vi "DWE Main3.vi"() -> ()   [LabVIEW 2014]
uses:
  TypeDefs/DWE Errors.ctl
  TypeDefs/DWE Data Info.ctl
  <vilib>/Utility/file.llb/Read From Spreadsheet File (string).vi
panel:
  out "Time array":timestamp[](array[timestamp])
  out "Cluster 2":T2
  out "Day":T2={"Info 1"={"Last time in range?"=TRUE, "Date"="", "Start index"=0}, "Info 2"={"Last time in range?"=TRUE, "Date"="", "Start index"=0}, "Info 3"={"Last time in range?"=TRUE, "Date"="", "Start index"=0}, "Info 4"={"Last time in range?"=TRUE, "Date"="", "Start index"=0}, "info 5"={"Last time in range?"=TRUE, "Date"="", "Start index"=0}, "Info 6"={"Last time in range?"=TRUE, "Date"="", "Start index"=0}, "Info 7"={"Last time in range?"=TRUE, "Date"="", "Start index"=0}, "Info 8"={"Last time in range?"=TRUE, "Date"="", "Start index"=0}, "Info 9"={"Last time in range?"=TRUE, "Date"="", "Start index"=0}, "Info 10"={"Last time in range?"=TRUE, "Date"="", "Start index"=0}}
  in  "Cluster":T2
  out "Iteration":i32
  out "ADC Count":dbl[](array[numeric])
  out "# of rows":i32
  in  "Tab Control":T3(tab)
  out "Current (mA)":cluster{dbl[], dbl[]}(graph)
  out "XY Graph 10":cluster{dbl[], dbl[]}[](graph)
  out "Digital signals":cluster{dbl[], dbl[]}[](graph)
  out "Errors 1":T4
  out "Current (mA) 2":cluster{dbl[], dbl[]}(graph)
  out "XY Graph 11":cluster{dbl[], dbl[]}[](graph)
  out "Digital signals 3":cluster{dbl[], dbl[]}[](graph)
  out "Errors 2":T4
  out "Digital signals 2":cluster{dbl[], dbl[]}[](graph)
  out "Current (mA) 3":cluster{dbl[], dbl[]}(graph)
  out "XY Graph 12":cluster{dbl[], dbl[]}[](graph)
  out "Errors 3":T4
  out "Digital signals 4":cluster{dbl[], dbl[]}[](graph)
  out "Current (mA) 4":cluster{dbl[], dbl[]}(graph)
  out "XY Graph 13":cluster{dbl[], dbl[]}[](graph)
  out "Errors 11":T4
  out "Digital signals 5":cluster{dbl[], dbl[]}[](graph)
  out "Current (mA) 5":cluster{dbl[], dbl[]}(graph)
  out "XY Graph 14":cluster{dbl[], dbl[]}[](graph)
  out "Errors 4":T4
  out "Digital signals 6":cluster{dbl[], dbl[]}[](graph)
  out "Current (mA) 6":cluster{dbl[], dbl[]}(graph)
  out "XY Graph 15":cluster{dbl[], dbl[]}[](graph)
  out "Errors 5":T4
  out "Digital signals 7":cluster{dbl[], dbl[]}[](graph)
  out "Current (mA) 7":cluster{dbl[], dbl[]}(graph)
  out "XY Graph 16":cluster{dbl[], dbl[]}[](graph)
  out "Errors 6":T4
  out "Digital signals 8":cluster{dbl[], dbl[]}[](graph)
  out "Current (mA) 8":cluster{dbl[], dbl[]}(graph)
  out "XY Graph 17":cluster{dbl[], dbl[]}[](graph)
  out "Errors 7":T4
  out "Digital signals 9":cluster{dbl[], dbl[]}[](graph)
  out "Current (mA) 9":cluster{dbl[], dbl[]}(graph)
  out "XY Graph 18":cluster{dbl[], dbl[]}[](graph)
  out "Errors 8":T4
  out "Digital signals 10":cluster{dbl[], dbl[]}[](graph)
  out "Current (mA) 10":cluster{dbl[], dbl[]}(graph)
  out "XY Graph 19":cluster{dbl[], dbl[]}[](graph)
  out "Errors 9":T4
  out "subarray":string[][](array[string])
  out "subarray 3":string[](array[string])
  in  "stop":bool
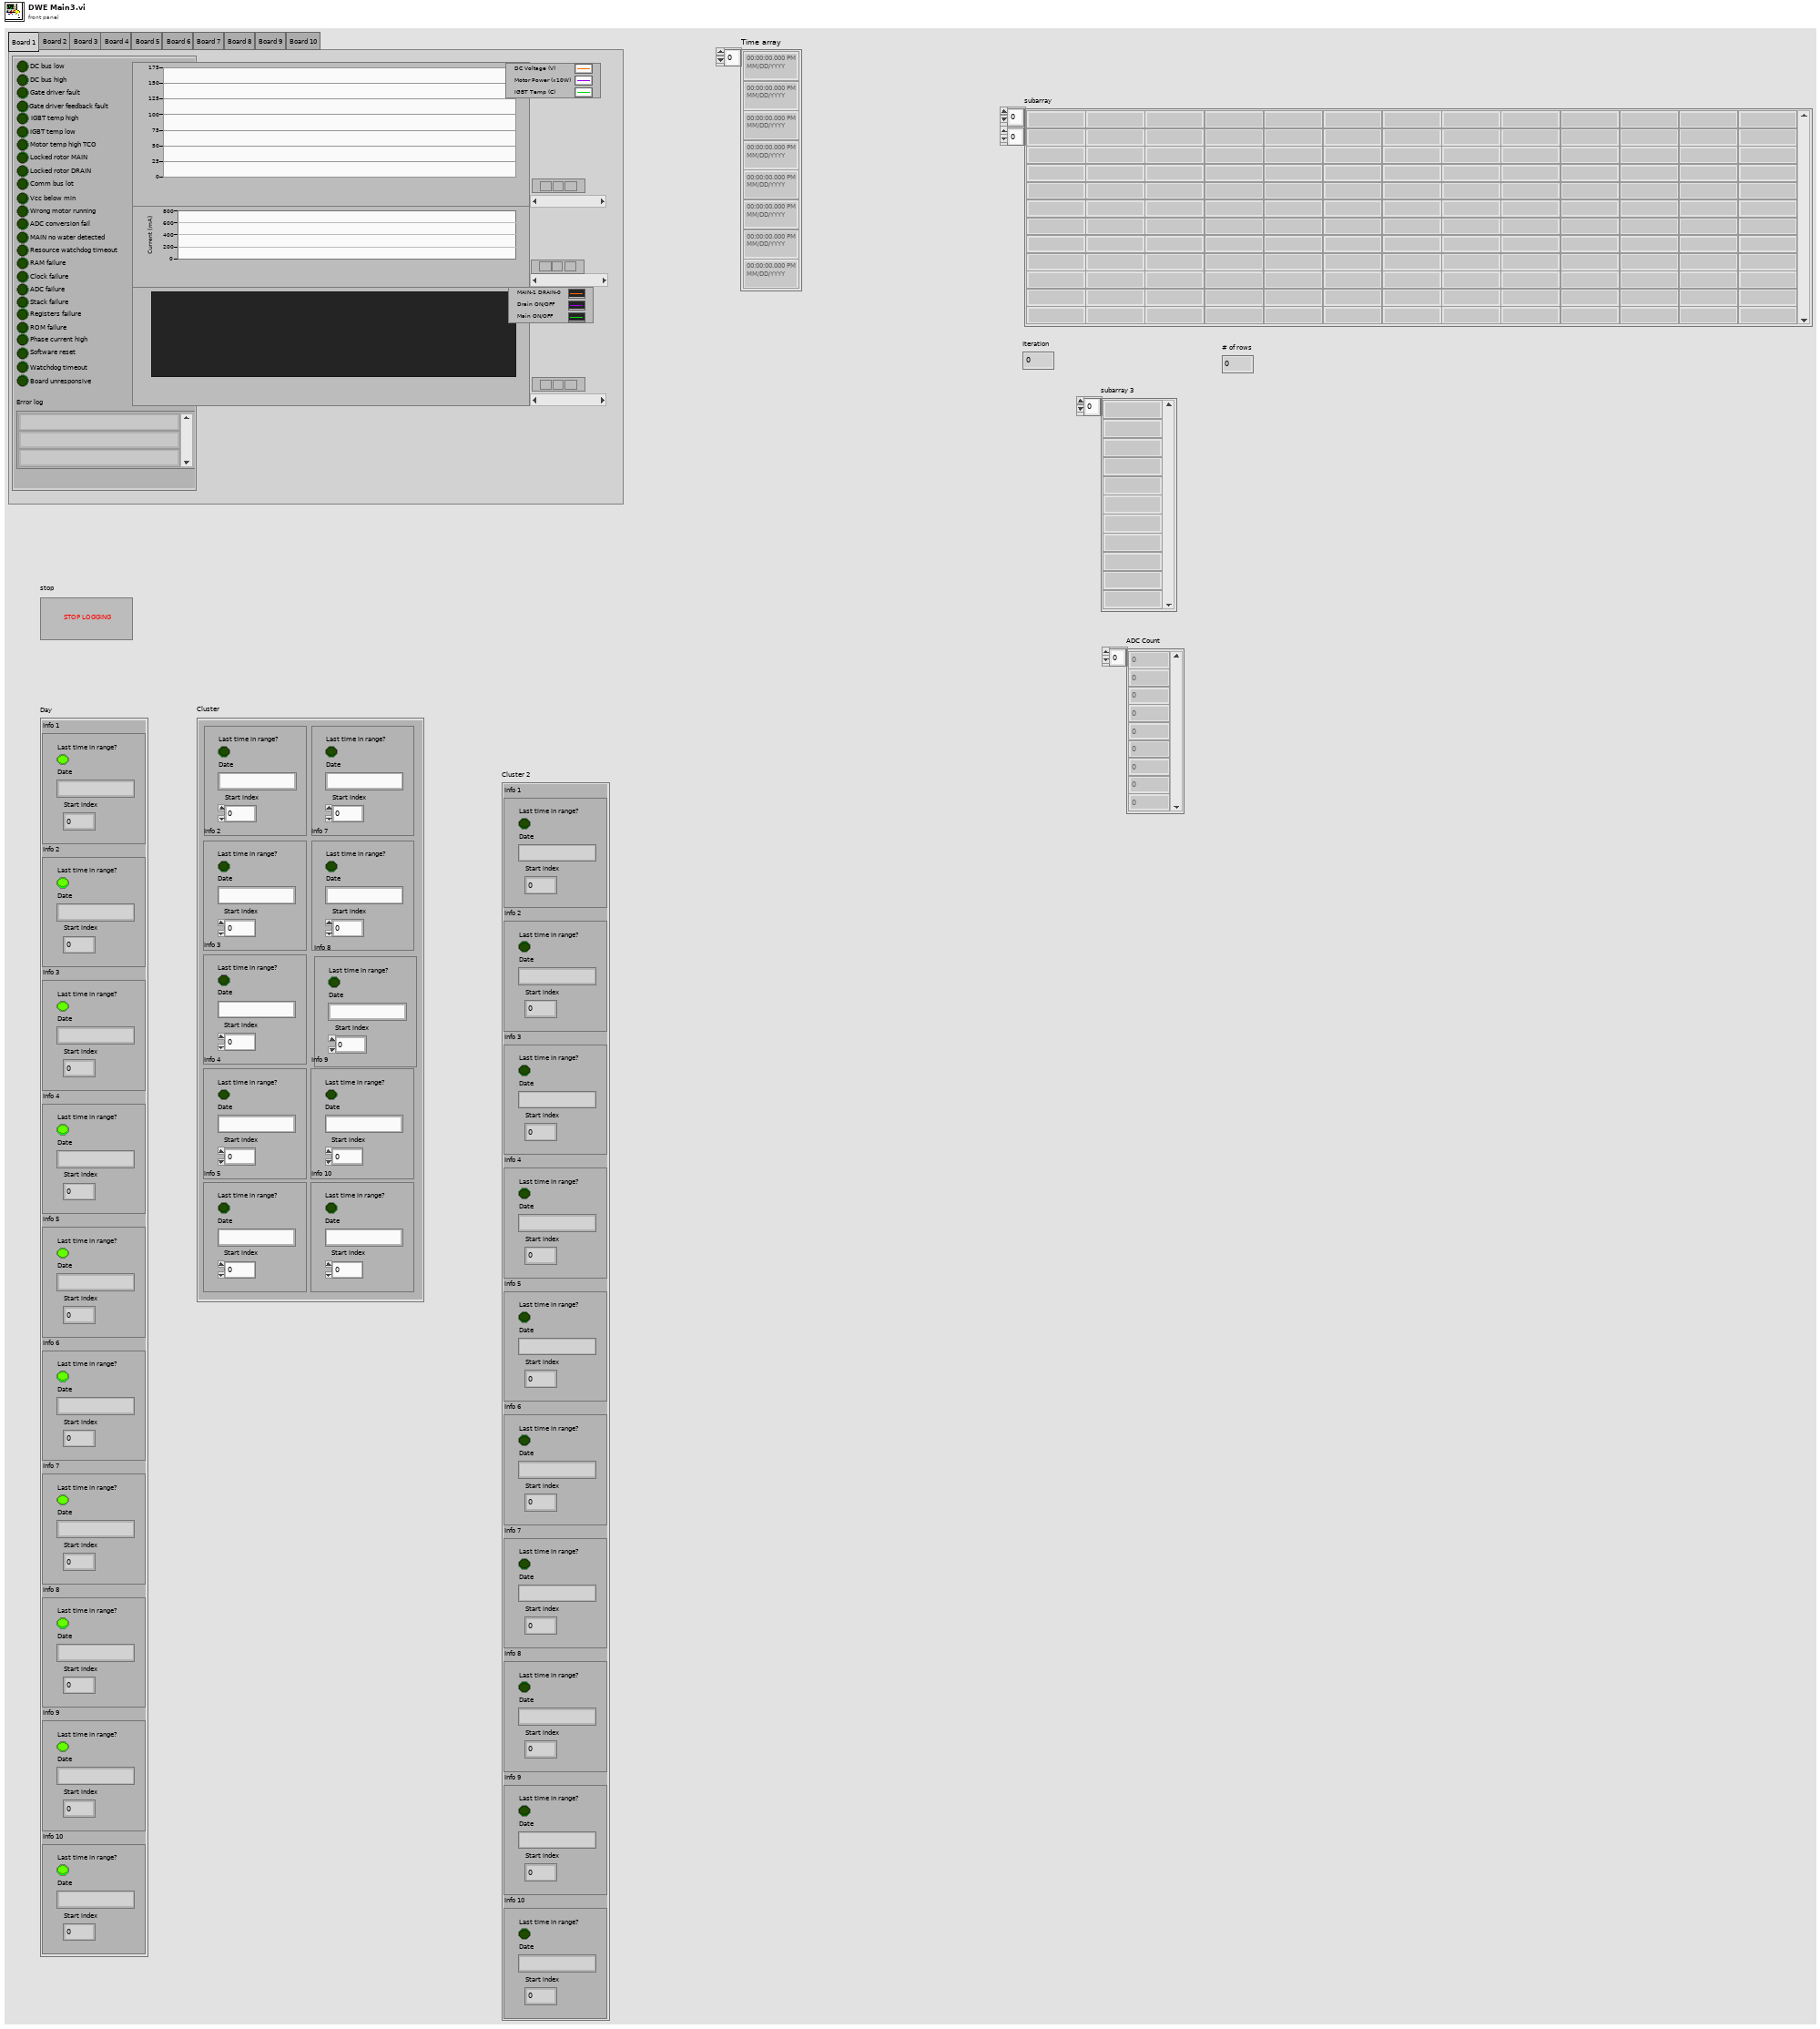
[diagram p1: front panel]
types:
  T1 = typedef "DWE Data Info.ctl" = cluster{"Last time in range?":bool, "Date":string, "Start index":i32}
  T2 = cluster{"Info 1":T1, "Info 2":T1, "Info 3":T1, "Info 4":T1, "info 5":T1, "Info 6":T1, "Info 7":T1, "Info 8":T1, "Info 9":T1, "Info 10":T1}
  T3 = enum32{"Board 1", "Board 2", "Board 3", "Board 4", "Board 5", "Board 6", "Board 7", "Board 8", "Board 9", "Board 10"}
  T4 = typedef "DWE Errors.ctl" = cluster{"DC bus low":bool, "DC bus high":bool, "Gate driver fault":bool, "Gate driver feedback fault":bool, "IGBT temp high":bool, "IGBT temp low":bool, "Motor temp high TCO":bool, "Locked rotor MAIN":bool, "Locked rotor DRAIN":bool, "Comm bus lot":bool, "Vcc below min":bool, "Wrong motor running":bool, "ADC conversion fail":bool, "MAIN no water detected":bool, "Resource watchdog timeout":bool, "RAM failure":bool, "Clock failure":bool, "ADC failure":bool, "Stack failure":bool, "Registers failure":bool, "ROM failure":bool, "Phase current high":bool, "Software reset":bool, "Watchdog timeout":bool, "Error log":string[], "Board unresponsive":bool}
  T5 = cluster{"01 File Path":path, "02 File Path":path, "03 File Path":path, "04 File Path":path, "05 File Path":path, "06 File Path":path, "07 File Path":path, "08 File Path":path, "09 File Path":path, "10 File Path":path}
  T6 = cluster{"Last time in range?":bool, "date/time string":string, "Start index":i32}
  T7 = cluster{"DC Bus Voltage":dbl, "Current RMS":dbl, "Motor Power":dbl, "IGBT Temp":u16, "Motor Type":u16, "Motor Power Sign":string, "Relay Position":u16, "ADC Count":dbl, "Recirculation Motor ON/OFF":u16, "Drain Motor ON/OFF":u16}
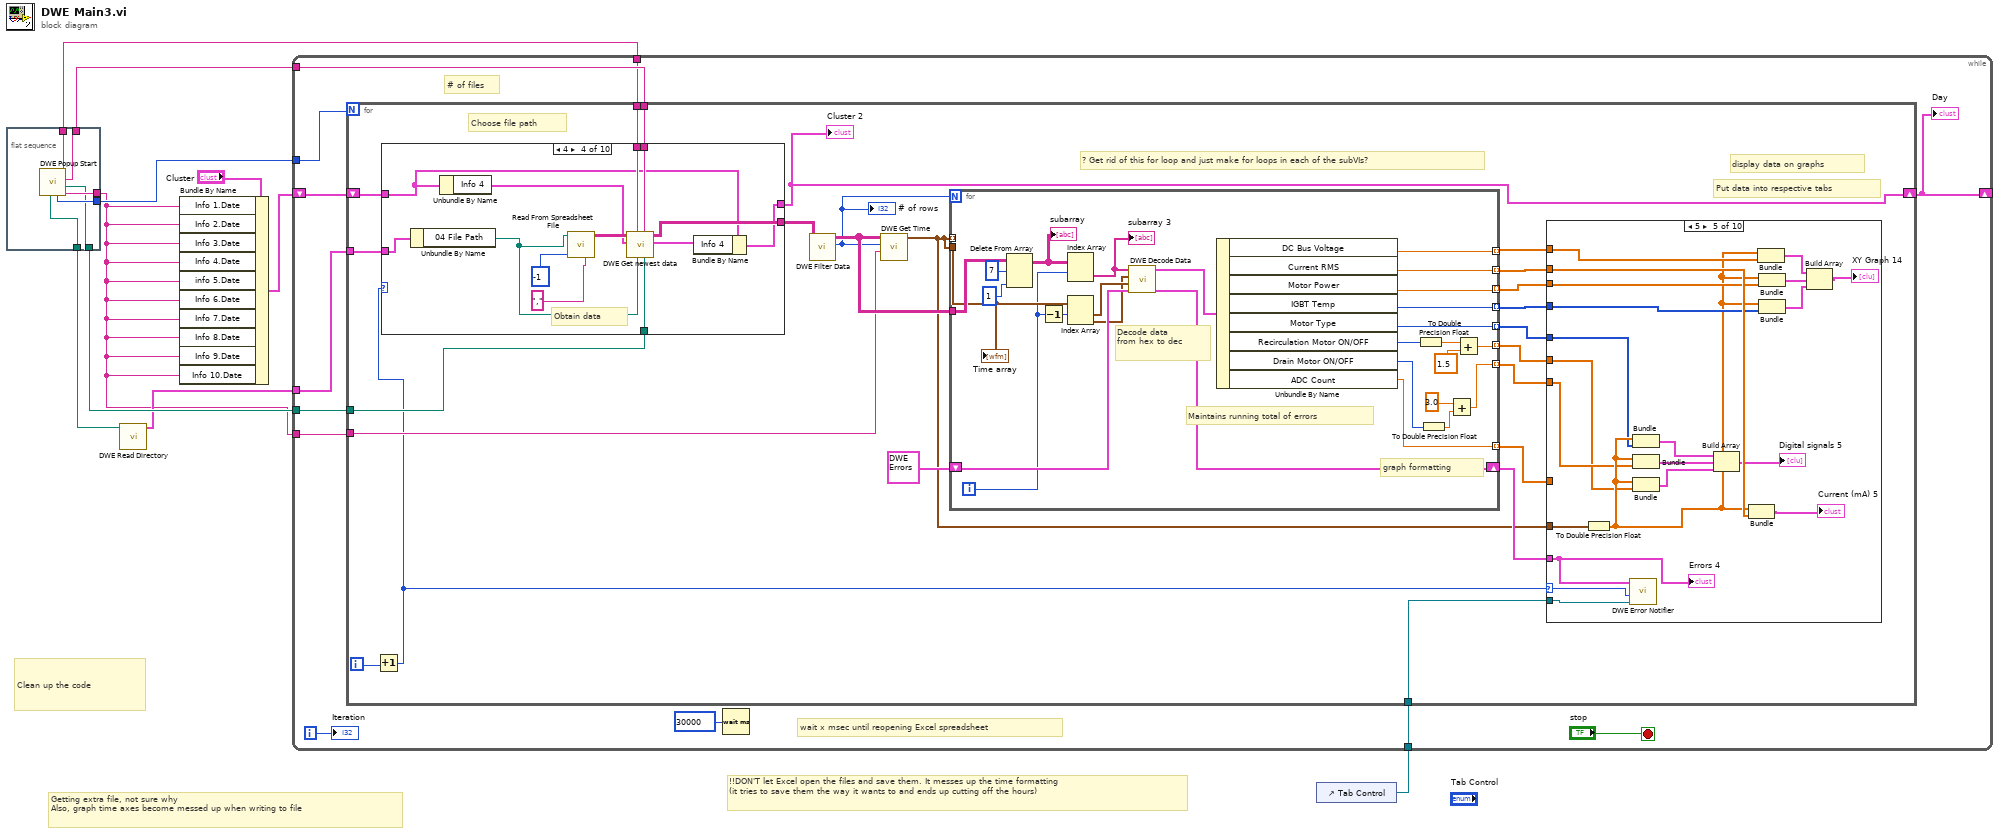
[diagram p0: block diagram]
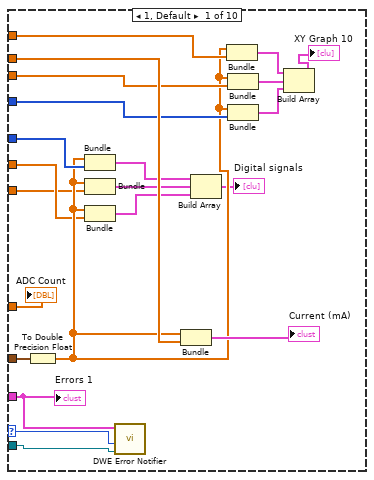
[diagram p2: hidden frame]
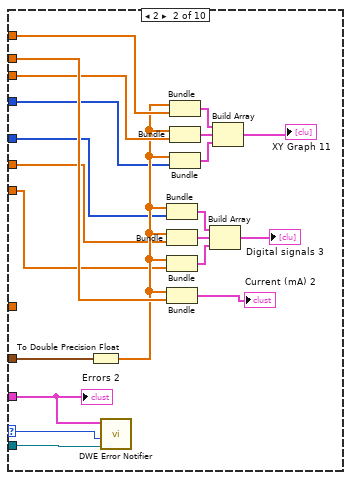
[diagram p3: hidden frame]
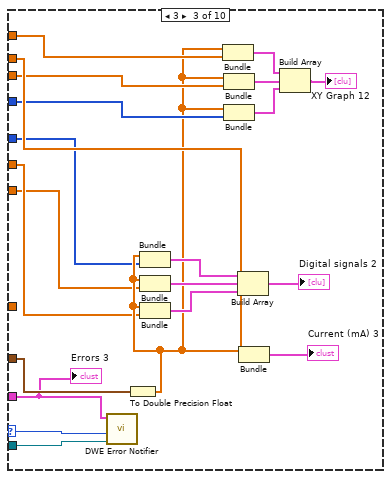
[diagram p4: hidden frame]
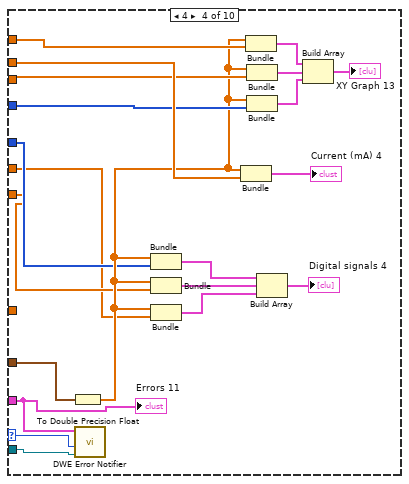
[diagram p5: hidden frame]
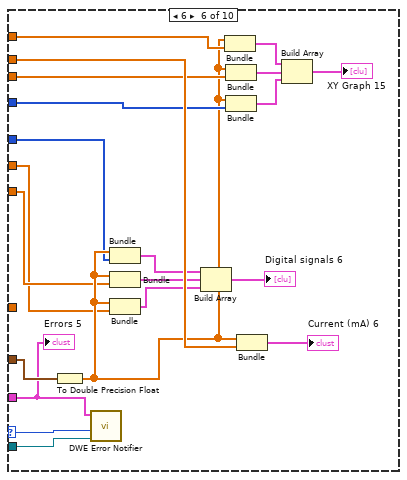
[diagram p6: hidden frame]
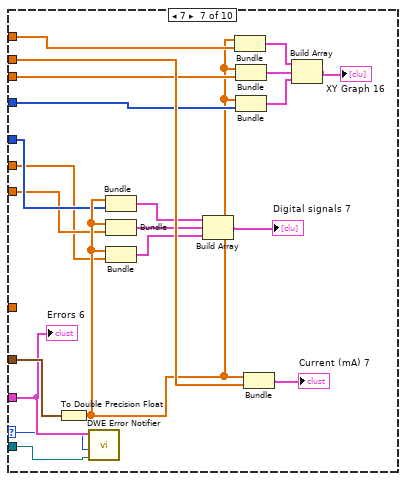
[diagram p7: hidden frame]
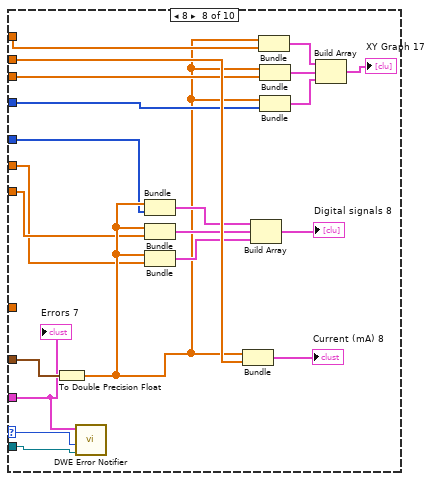
[diagram p8: hidden frame]
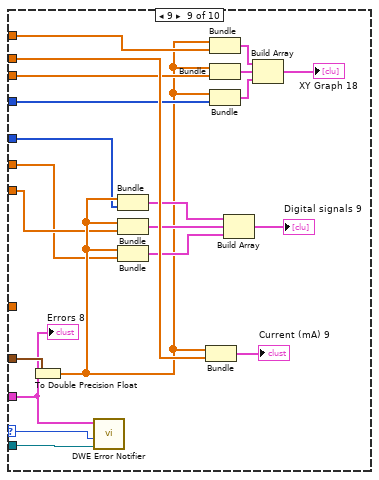
[diagram p9: hidden frame]
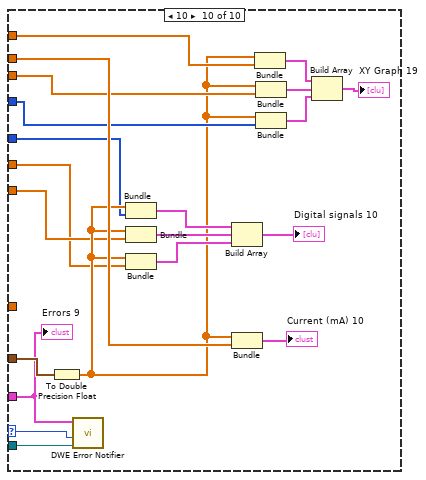
[diagram p10: hidden frame]
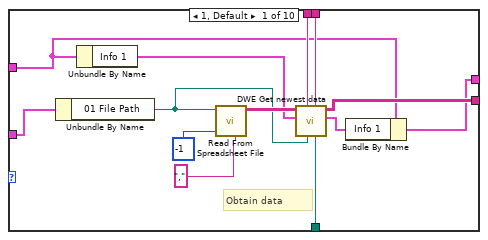
[diagram p11: hidden frame]
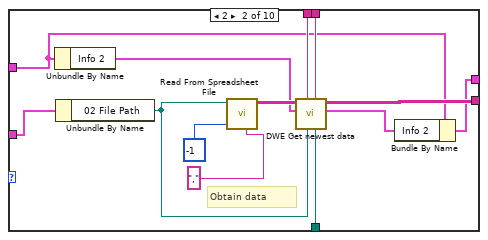
[diagram p12: hidden frame]
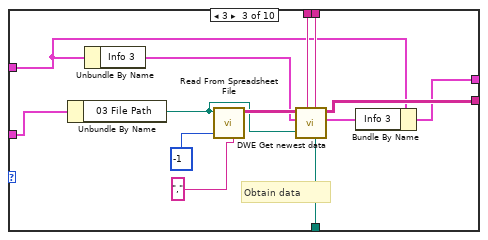
[diagram p13: hidden frame]
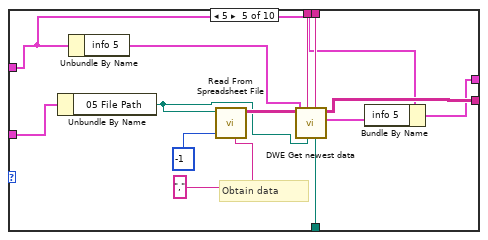
[diagram p14: hidden frame]
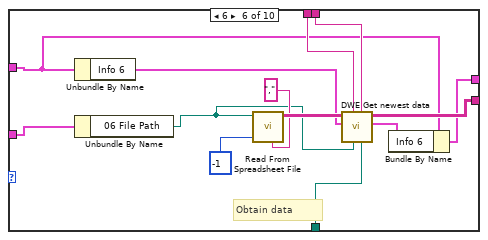
[diagram p15: hidden frame]
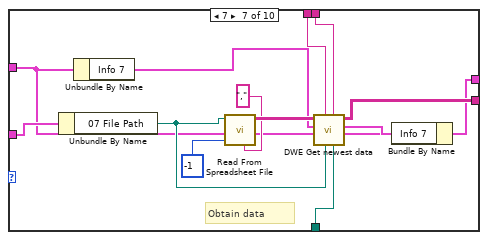
[diagram p16: hidden frame]
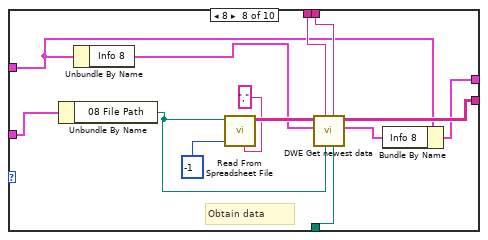
[diagram p17: hidden frame]
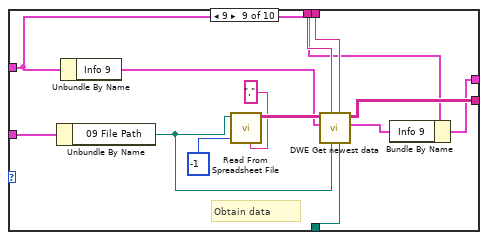
[diagram p18: hidden frame]
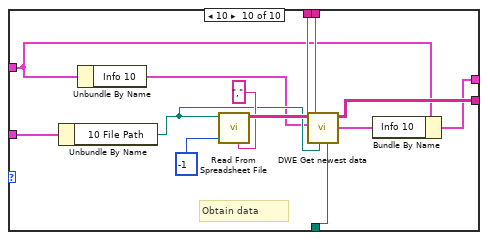
[diagram p19: hidden frame]
diagram:
  # "Getting extra file, not sure why\nAlso, graph time axes become messed up when writing to file"
  # "Clean up the code"
  # "!!DON'T let Excel open the files and save them. It messes up the time formatting \n(it tries to save them the way it wants to and ends up cutting off the hours)"
  n1 = flat-sequence {
    tunnel: [w16] -> w2
    tunnel: [w15] -> w8
    tunnel: [w14] -> w3
    tunnel: [w13] -> w7
    tunnel: [w12] -> w6
    tunnel: [w11] -> w5
    frame #0 {
      n2 = call "DWE Popup Start.vi"() -> ("Date Laundry.NET\nstarted (MM_DD) 2"=w16:string, "Folder to store data sets 2"=w13:path, "End time save 2"=w12:string, "Start time save 2"=w11:string, "# of Files 2"=w15:i32, "File directory 2"=w14:path)  [unwired: 6 in]
    }
  }
  n3 = call "DWE Read Directory.vi"("path"=w3) -> ("Laundry.NET \nfile paths 3"=w4:T5)  [unwired: 10 in]
  n4 = Bundle By Name(cluster="Cluster", "Info 1.Date"=w2, "Info 2.Date"=w2, "Info 3.Date"=w2, "Info 4.Date"=w2, "info 5.Date"=w2, "Info 6.Date"=w2, "Info 7.Date"=w2, "Info 8.Date"=w2, "Info 9.Date"=w2, "Info 10.Date"=w2) -> (w9:T2)
  n5 = control-ref of="Tab Control"() -> (w1:refnum<vi>)
  n6 = while {
    shift-right: [w25] -> _
    shift-left: w9 -> [w19]
    tunnel: w8 -> [w24]
    tunnel: w4 -> [w23]
    tunnel: w7 -> [w22]
    tunnel: w6 -> [w21]
    tunnel: w5 -> [w20]
    tunnel: w2 -> [w18]
    tunnel: w1 -> [w17]
    i -> [w26]
    stop <- "stop" stop-if-true
    # "# of files"
    # "wait x msec until reopening Excel spreadsheet"
    n7 = for {
      N: w24 -> [_]
      tunnel: w23 -> [w52]
      tunnel: w21 -> [w39]
      tunnel: w22 -> [w37]
      tunnel: w20 -> [w36]
      shift-right: [w38] -> w25
      shift-left: w19 -> [w35]
      tunnel: w18 -> [w33]
      tunnel: w17 -> [w32]
      i -> [w31]
      # "? Get rid of this for loop and just make for loops in each of the subVIs?"
      # "display data on graphs"
      # "Put data into respective tabs"
      # "Choose file path"
      n8 = Increment(x=w31) -> (x+1=w30:i32)
      n9 = case shown="4" w30 {
        tunnel: w52 -> [w276 w289 w302 w315 w328 w341 w354 w367 w380 w393]
        tunnel: [w272 w285 w298 w311 w324 w337 w350 w363 w376 w389] -> w40
        tunnel: w37 -> [w270 w281 w294 w307 w320 w335 w346 w359 w372 w385]
        tunnel: w36 -> [w269 w284 w297 w310 w323 w334 w349 w362 w375 w388]
        tunnel: w39 -> [w268 w283 w296 w309 w322 w333 w348 w361 w374 w387]
        tunnel: w35 -> [w265 w278 w292 w304 w317 w330 w343 w356 w369 w383]
        tunnel: [w264 w277 w290 w303 w316 w329 w342 w355 w368 w381] -> w38
        frame 1, Default {
          # "Obtain data"
          n10 = Unbundle By Name(w276) -> ("01 File Path"=w271:path)
          n11 = Unbundle By Name(w265) -> ("Info 1"=w267:T1)
          n12 = call-poly <vilib>:"Read From Spreadsheet File.vi"("delimiter (\\t)"="," ("delimiter (\\t)"), "number of rows (all:-1)"=-1, "file path (dialog if empty)"=w271) -> ("all rows"=w275:string[][])  [unwired: 4 in, 4 out]
          n13 = call "DWE Get newest data.vi"("target path"=w270, "End time"=w268, "source path"=w271, "Start time"=w269, "Previous info"=w267, "all rows"=w275) -> ("New Info"=w266:T6, "newest rows"=w272:string[][])  [unwired: 4 in]
          n14 = Bundle By Name(cluster=w265, "Info 1"=w266) -> (w264:T2)
        }
        frame 2 {
          # "Obtain data"
          n15 = Unbundle By Name(w278) -> ("Info 2"=w280:T1)
          n16 = Unbundle By Name(w289) -> ("02 File Path"=w282:path)
          n17 = call-poly <vilib>:"Read From Spreadsheet File.vi"("delimiter (\\t)"="," ("delimiter (\\t)"), "number of rows (all:-1)"=-1, "file path (dialog if empty)"=w282) -> ("all rows"=w288:string[][])  [unwired: 4 in, 4 out]
          n18 = call "DWE Get newest data.vi"("target path"=w281, "End time"=w283, "source path"=w282, "Start time"=w284, "Previous info"=w280, "all rows"=w288) -> ("New Info"=w279:T6, "newest rows"=w285:string[][])  [unwired: 4 in]
          n19 = Bundle By Name(cluster=w278, "Info 2"=w279) -> (w277:T2)
        }
        frame 3 {
          # "Obtain data"
          n20 = Unbundle By Name(w302) -> ("03 File Path"=w295:path)
          n21 = Unbundle By Name(w292) -> ("Info 3"=w293:T1)
          n22 = call-poly <vilib>:"Read From Spreadsheet File.vi"("delimiter (\\t)"="," ("delimiter (\\t)"), "number of rows (all:-1)"=-1, "file path (dialog if empty)"=w295) -> ("all rows"=w301:string[][])  [unwired: 4 in, 4 out]
          n23 = call "DWE Get newest data.vi"("target path"=w294, "End time"=w296, "source path"=w295, "Start time"=w297, "Previous info"=w293, "all rows"=w301) -> ("New Info"=w291:T6, "newest rows"=w298:string[][])  [unwired: 4 in]
          n24 = Bundle By Name(cluster=w292, "Info 3"=w291) -> (w290:T2)
        }
        frame 4 {
          # "Obtain data"
          n25 = Unbundle By Name(w315) -> ("04 File Path"=w308:path)
          n26 = Unbundle By Name(w304) -> ("Info 4"=w306:T1)
          n27 = call-poly <vilib>:"Read From Spreadsheet File.vi"("delimiter (\\t)"="," ("delimiter (\\t)"), "number of rows (all:-1)"=-1, "file path (dialog if empty)"=w308) -> ("all rows"=w314:string[][])  [unwired: 4 in, 4 out]
          n28 = call "DWE Get newest data.vi"("target path"=w307, "End time"=w309, "source path"=w308, "Start time"=w310, "Previous info"=w306, "all rows"=w314) -> ("New Info"=w305:T6, "newest rows"=w311:string[][])  [unwired: 4 in]
          n29 = Bundle By Name(cluster=w304, "Info 4"=w305) -> (w303:T2)
        }
        frame 5 {
          # "Obtain data"
          n30 = Unbundle By Name(w328) -> ("05 File Path"=w321:path)
          n31 = Unbundle By Name(w317) -> ("info 5"=w319:T1)
          n32 = call-poly <vilib>:"Read From Spreadsheet File.vi"("delimiter (\\t)"="," ("delimiter (\\t)"), "number of rows (all:-1)"=-1, "file path (dialog if empty)"=w321) -> ("all rows"=w327:string[][])  [unwired: 4 in, 4 out]
          n33 = call "DWE Get newest data.vi"("target path"=w320, "End time"=w322, "source path"=w321, "Start time"=w323, "Previous info"=w319, "all rows"=w327) -> ("New Info"=w318:T6, "newest rows"=w324:string[][])  [unwired: 4 in]
          n34 = Bundle By Name(cluster=w317, "info 5"=w318) -> (w316:T2)
        }
        frame 6 {
          # "Obtain data"
          n35 = Unbundle By Name(w330) -> ("Info 6"=w332:T1)
          n36 = Unbundle By Name(w341) -> ("06 File Path"=w336:path)
          n37 = call-poly <vilib>:"Read From Spreadsheet File.vi"("delimiter (\\t)"="," ("delimiter (\\t)"), "number of rows (all:-1)"=-1, "file path (dialog if empty)"=w336) -> ("all rows"=w340:string[][])  [unwired: 4 in, 4 out]
          n38 = call "DWE Get newest data.vi"("target path"=w335, "End time"=w333, "source path"=w336, "Start time"=w334, "Previous info"=w332, "all rows"=w340) -> ("New Info"=w331:T6, "newest rows"=w337:string[][])  [unwired: 4 in]
          n39 = Bundle By Name(cluster=w330, "Info 6"=w331) -> (w329:T2)
        }
        frame 7 {
          # "Obtain data"
          n40 = Unbundle By Name(w354) -> ("07 File Path"=w347:path)
          n41 = Unbundle By Name(w343) -> ("Info 7"=w345:T1)
          n42 = call-poly <vilib>:"Read From Spreadsheet File.vi"("delimiter (\\t)"="," ("delimiter (\\t)"), "number of rows (all:-1)"=-1, "file path (dialog if empty)"=w347) -> ("all rows"=w353:string[][])  [unwired: 4 in, 4 out]
          n43 = call "DWE Get newest data.vi"("target path"=w346, "End time"=w348, "source path"=w347, "Start time"=w349, "Previous info"=w345, "all rows"=w353) -> ("New Info"=w344:T6, "newest rows"=w350:string[][])  [unwired: 4 in]
          n44 = Bundle By Name(cluster=w343, "Info 7"=w344) -> (w342:T2)
        }
        frame 8 {
          # "Obtain data"
          n45 = Unbundle By Name(w367) -> ("08 File Path"=w360:path)
          n46 = Unbundle By Name(w356) -> ("Info 8"=w358:T1)
          n47 = call-poly <vilib>:"Read From Spreadsheet File.vi"("delimiter (\\t)"="," ("delimiter (\\t)"), "number of rows (all:-1)"=-1, "file path (dialog if empty)"=w360) -> ("all rows"=w366:string[][])  [unwired: 4 in, 4 out]
          n48 = call "DWE Get newest data.vi"("target path"=w359, "End time"=w361, "source path"=w360, "Start time"=w362, "Previous info"=w358, "all rows"=w366) -> ("New Info"=w357:T6, "newest rows"=w363:string[][])  [unwired: 4 in]
          n49 = Bundle By Name(cluster=w356, "Info 8"=w357) -> (w355:T2)
        }
        frame 9 {
          # "Obtain data"
          n50 = Unbundle By Name(w380) -> ("09 File Path"=w373:path)
          n51 = Unbundle By Name(w369) -> ("Info 9"=w371:T1)
          n52 = call-poly <vilib>:"Read From Spreadsheet File.vi"("delimiter (\\t)"="," ("delimiter (\\t)"), "number of rows (all:-1)"=-1, "file path (dialog if empty)"=w373) -> ("all rows"=w379:string[][])  [unwired: 4 in, 4 out]
          n53 = call "DWE Get newest data.vi"("target path"=w372, "End time"=w374, "source path"=w373, "Start time"=w375, "Previous info"=w371, "all rows"=w379) -> ("New Info"=w370:T6, "newest rows"=w376:string[][])  [unwired: 4 in]
          n54 = Bundle By Name(cluster=w369, "Info 9"=w370) -> (w368:T2)
        }
        frame 10 {
          # "Obtain data"
          n55 = Unbundle By Name(w393) -> ("10 File Path"=w386:path)
          n56 = Unbundle By Name(w383) -> ("Info 10"=w384:T1)
          n57 = call-poly <vilib>:"Read From Spreadsheet File.vi"("delimiter (\\t)"="," ("delimiter (\\t)"), "number of rows (all:-1)"=-1, "file path (dialog if empty)"=w386) -> ("all rows"=w392:string[][])  [unwired: 4 in, 4 out]
          n58 = call "DWE Get newest data.vi"("target path"=w385, "End time"=w387, "source path"=w386, "Start time"=w388, "Previous info"=w384, "all rows"=w392) -> ("New Info"=w382:T6, "newest rows"=w389:string[][])  [unwired: 4 in]
          n59 = Bundle By Name(cluster=w383, "Info 10"=w382) -> (w381:T2)
        }
      }
      "Cluster 2" <- w38
      n60 = call "DWE Filter Data.vi"("All Rows"=w40) -> ("element"=w34:i32, "new array"=w45:string[][])  [unwired: 9 in]
      "# of rows" <- w34
      n61 = call "DWE Get Time.vi"("Date"=w33, "# of rows"=w34, "Data row"=w45) -> ("Time array"=w29:timestamp[])  [unwired: 8 in]
      n62 = for {
        N: w34 -> [_]
        tunnel: [w420] -> w49 mode=indexing
        tunnel: [w419] -> w51 mode=indexing
        tunnel: [w418] -> w50 mode=indexing
        tunnel: [w417] -> w48 mode=indexing
        tunnel: [w416] -> w47 mode=indexing
        shift-right: [w403] -> w46
        shift-left: T4 {"DC bus low"=FALSE, "DC bus high"=FALSE, "Gate driver fault"=FALSE, "Gate driver feedback fault"=FALSE, "IGBT temp high"=FALSE, "IGBT temp low"=FALSE, "Motor temp high TCO"=FALSE, "Locked rotor MAIN"=FALSE, "Locked rotor DRAIN"=FALSE, "Comm bus lot"=FALSE, "Vcc below min"=FALSE, "Wrong motor running"=FALSE, "ADC conversion fail"=FALSE, "MAIN no water detected"=FALSE, "Resource watchdog timeout"=FALSE, "RAM failure"=FALSE, "Clock failure"=FALSE, "ADC failure"=FALSE, "Stack failure"=FALSE, "Registers failure"=FALSE, "ROM failure"=FALSE, "Phase current high"=FALSE, "Software reset"=FALSE, "Watchdog timeout"=FALSE, "Error log"=[], "Board unresponsive"=FALSE} ("Errors Out") -> [w415]
        tunnel: w45 -> [w402]
        tunnel: [w412] -> w42 mode=indexing
        tunnel: [w411] -> w43 mode=indexing
        tunnel: [w404] -> w41 mode=indexing
        tunnel: w29 -> [_] mode=indexing
        tunnel: w29 -> [w398]
        i -> [w394]
        # "graph formatting"
        # "Maintains running total of errors"
        # "Decode data\nfrom hex to dec"
        n63 = Delete From Array(array=w402, length=7, index (col)=1 ("disabled index (col)")) -> (array with subset deleted=w399:string[][])  [unwired: 1 in, 1 out]
        "subarray" <- w399
        n64 = Decrement(x=w394) -> (x-1=w395:i32)
        n65 = Index Array(array=w399, index (row)=w394) -> (element=w413:string[])  [unwired: 1 in]
        "subarray 3" <- w413
        n66 = Index Array(array=w398, index #1=w395) -> (element #1=w397:timestamp, element #2=w396:timestamp)  [unwired: 1 in]
        n67 = call "DWE Decode Data.vi"("Errors In"=w415, "Prev time stamp"=w397, "Time Stamp"=w396, "Data Array"=w413) -> ("Errors Out"=w403:T4, "logData Out"=w414:T7)  [unwired: 6 in]
        n68 = Unbundle By Name(w414) -> ("DC Bus Voltage"=w420:dbl, "Current RMS"=w419:dbl, "Motor Power"=w418:dbl, "IGBT Temp"=w417:u16, "Motor Type"=w416:u16, "Recirculation Motor ON/OFF"=w410:u16, "Drain Motor ON/OFF"=w407:u16, "ADC Count"=w404:dbl)
        n69 = To Double Precision Float(number=w410) -> (double precision float=w409:dbl)
        n70 = To Double Precision Float(number=w407) -> (double precision float=w406:dbl)
        n71 = Add(x=3.0, y=w406) -> (x+y=w411:dbl)
        n72 = Add(x=w409, y=1.5) -> (x+y=w412:dbl)
        "Time array" <- w398
      }
      n73 = case shown="5" w30 {
        selector: w30 -> [w54 w76 w97 w118 w140 w160 w181 w202 w223 w244]
        tunnel: w51 -> [w74 w94 w115 w136 w157 w178 w199 w220 w241 w262]
        tunnel: w50 -> [w66 w89 w110 w130 w152 w173 w194 w215 w237 w260]
        tunnel: w49 -> [w67 w90 w111 w132 w153 w174 w195 w216 w238 w261]
        tunnel: w48 -> [w65 w84 w109 w131 w151 w172 w193 w214 w236 w259]
        tunnel: w47 -> [w64 w78 w104 w125 w146 w167 w188 w209 w230 w251]
        tunnel: w46 -> [w55 w77 w98 w119 w141 w161 w182 w203 w224 w245]
        tunnel: w29 -> [w73 w95 w116 w137 w158 w179 w200 w221 w242 w263]
        tunnel: w42 -> [w62 w83 w103 w123 w144 w165 w186 w207 w228 w249]
        tunnel: w43 -> [w61 w82 w102 w124 w145 w166 w187 w208 w229 w250]
        tunnel: w41 -> [w56 _ _ _ _ _ _ _ _ _]
        tunnel: w32 -> [w53 w75 w96 w117 w139 w159 w180 w201 w222 w243]
        frame 1, Default {
          n74 = To Double Precision Float(number=w73) -> (double precision float=w63:dbl[])
          n75 = Bundle(w63, w64) -> (w60:cluster{dbl[], u16[]})  [unwired: 1 in]
          n76 = Bundle(w63, w61) -> (w58:cluster{dbl[], dbl[]})  [unwired: 1 in]
          n77 = Bundle(w63, w62) -> (w57:cluster{dbl[], dbl[]})  [unwired: 1 in]
          n78 = call "DWE Error Notifier.vi"("Tab Control 3"=w53, "Tab num"=w54, "Errors 1"=w55) -> ()  [unwired: 8 in, 1 out]
          n79 = Bundle(w63, w74) -> (→"Current (mA)":cluster{dbl[], dbl[]})  [unwired: 1 in]
          n80 = Build Array(w60, w58, w57) -> (→"Digital signals":cluster{dbl[], dbl[]}[])
          n81 = Bundle(w63, w67) -> (w71:cluster{dbl[], dbl[]})  [unwired: 1 in]
          n82 = Bundle(w63, w66) -> (w70:cluster{dbl[], dbl[]})  [unwired: 1 in]
          n83 = Bundle(w63, w65) -> (w69:cluster{dbl[], u16[]})  [unwired: 1 in]
          n84 = Build Array(w71, w70, w69) -> (→"XY Graph 10":cluster{dbl[], dbl[]}[])
          "Errors 1" <- w55
          "ADC Count" <- w56
        }
        frame 2 {
          n85 = To Double Precision Float(number=w95) -> (double precision float=w85:dbl[])
          n86 = call "DWE Error Notifier.vi"("Tab Control 3"=w75, "Tab num"=w76, "Errors 1"=w77) -> ()  [unwired: 8 in, 1 out]
          n87 = Bundle(w85, w78) -> (w88:cluster{dbl[], u16[]})  [unwired: 1 in]
          n88 = Bundle(w85, w83) -> (w87:cluster{dbl[], dbl[]})  [unwired: 1 in]
          n89 = Bundle(w85, w82) -> (w86:cluster{dbl[], dbl[]})  [unwired: 1 in]
          n90 = Bundle(w85, w94) -> (→"Current (mA) 2":cluster{dbl[], dbl[]})  [unwired: 1 in]
          n91 = Bundle(w85, w90) -> (w93:cluster{dbl[], dbl[]})  [unwired: 1 in]
          n92 = Bundle(w85, w89) -> (w92:cluster{dbl[], dbl[]})  [unwired: 1 in]
          n93 = Bundle(w85, w84) -> (w91:cluster{dbl[], u16[]})  [unwired: 1 in]
          n94 = Build Array(w88, w87, w86) -> (→"Digital signals 3":cluster{dbl[], dbl[]}[])
          n95 = Build Array(w93, w92, w91) -> (→"XY Graph 11":cluster{dbl[], dbl[]}[])
          "Errors 2" <- w77
        }
        frame 3 {
          n96 = call "DWE Error Notifier.vi"("Tab Control 3"=w96, "Tab num"=w97, "Errors 1"=w98) -> ()  [unwired: 8 in, 1 out]
          n97 = To Double Precision Float(number=w116) -> (double precision float=w105:dbl[])
          n98 = Bundle(w105, w104) -> (w108:cluster{dbl[], u16[]})  [unwired: 1 in]
          n99 = Bundle(w105, w102) -> (w107:cluster{dbl[], dbl[]})  [unwired: 1 in]
          n100 = Bundle(w105, w103) -> (w106:cluster{dbl[], dbl[]})  [unwired: 1 in]
          n101 = Bundle(w105, w111) -> (w114:cluster{dbl[], dbl[]})  [unwired: 1 in]
          n102 = Bundle(w105, w110) -> (w113:cluster{dbl[], dbl[]})  [unwired: 1 in]
          n103 = Bundle(w105, w109) -> (w112:cluster{dbl[], u16[]})  [unwired: 1 in]
          n104 = Build Array(w108, w107, w106) -> (→"Digital signals 2":cluster{dbl[], dbl[]}[])
          n105 = Bundle(w105, w115) -> (→"Current (mA) 3":cluster{dbl[], dbl[]})  [unwired: 1 in]
          n106 = Build Array(w114, w113, w112) -> (→"XY Graph 12":cluster{dbl[], dbl[]}[])
          "Errors 3" <- w98
        }
        frame 4 {
          n107 = To Double Precision Float(number=w137) -> (double precision float=w126:dbl[])
          n108 = call "DWE Error Notifier.vi"("Tab Control 3"=w117, "Tab num"=w118, "Errors 1"=w119) -> ()  [unwired: 8 in, 1 out]
          n109 = Bundle(w126, w125) -> (w129:cluster{dbl[], u16[]})  [unwired: 1 in]
          n110 = Bundle(w126, w124) -> (w128:cluster{dbl[], dbl[]})  [unwired: 1 in]
          n111 = Bundle(w126, w123) -> (w127:cluster{dbl[], dbl[]})  [unwired: 1 in]
          n112 = Bundle(w126, w136) -> (→"Current (mA) 4":cluster{dbl[], dbl[]})  [unwired: 1 in]
          n113 = Bundle(w126, w132) -> (w135:cluster{dbl[], dbl[]})  [unwired: 1 in]
          n114 = Bundle(w126, w130) -> (w134:cluster{dbl[], dbl[]})  [unwired: 1 in]
          n115 = Bundle(w126, w131) -> (w133:cluster{dbl[], u16[]})  [unwired: 1 in]
          n116 = Build Array(w129, w128, w127) -> (→"Digital signals 4":cluster{dbl[], dbl[]}[])
          n117 = Build Array(w135, w134, w133) -> (→"XY Graph 13":cluster{dbl[], dbl[]}[])
          "Errors 11" <- w119
        }
        frame 5 {
          n118 = To Double Precision Float(number=w158) -> (double precision float=w147:dbl[])
          n119 = call "DWE Error Notifier.vi"("Tab Control 3"=w139, "Tab num"=w140, "Errors 1"=w141) -> ()  [unwired: 8 in, 1 out]
          n120 = Bundle(w147, w146) -> (w150:cluster{dbl[], u16[]})  [unwired: 1 in]
          n121 = Bundle(w147, w145) -> (w149:cluster{dbl[], dbl[]})  [unwired: 1 in]
          n122 = Bundle(w147, w144) -> (w148:cluster{dbl[], dbl[]})  [unwired: 1 in]
          n123 = Build Array(w150, w149, w148) -> (→"Digital signals 5":cluster{dbl[], dbl[]}[])
          n124 = Bundle(w147, w157) -> (→"Current (mA) 5":cluster{dbl[], dbl[]})  [unwired: 1 in]
          n125 = Bundle(w147, w153) -> (w156:cluster{dbl[], dbl[]})  [unwired: 1 in]
          n126 = Bundle(w147, w152) -> (w155:cluster{dbl[], dbl[]})  [unwired: 1 in]
          n127 = Bundle(w147, w151) -> (w154:cluster{dbl[], u16[]})  [unwired: 1 in]
          n128 = Build Array(w156, w155, w154) -> (→"XY Graph 14":cluster{dbl[], dbl[]}[])
          "Errors 4" <- w141
        }
        frame 6 {
          n129 = To Double Precision Float(number=w179) -> (double precision float=w168:dbl[])
          n130 = call "DWE Error Notifier.vi"("Tab Control 3"=w159, "Tab num"=w160, "Errors 1"=w161) -> ()  [unwired: 8 in, 1 out]
          n131 = Bundle(w168, w167) -> (w171:cluster{dbl[], u16[]})  [unwired: 1 in]
          n132 = Bundle(w168, w166) -> (w170:cluster{dbl[], dbl[]})  [unwired: 1 in]
          n133 = Bundle(w168, w165) -> (w169:cluster{dbl[], dbl[]})  [unwired: 1 in]
          n134 = Build Array(w171, w170, w169) -> (→"Digital signals 6":cluster{dbl[], dbl[]}[])
          n135 = Bundle(w168, w174) -> (w177:cluster{dbl[], dbl[]})  [unwired: 1 in]
          n136 = Bundle(w168, w173) -> (w176:cluster{dbl[], dbl[]})  [unwired: 1 in]
          n137 = Bundle(w168, w172) -> (w175:cluster{dbl[], u16[]})  [unwired: 1 in]
          n138 = Bundle(w168, w178) -> (→"Current (mA) 6":cluster{dbl[], dbl[]})  [unwired: 1 in]
          n139 = Build Array(w177, w176, w175) -> (→"XY Graph 15":cluster{dbl[], dbl[]}[])
          "Errors 5" <- w161
        }
        frame 7 {
          n140 = To Double Precision Float(number=w200) -> (double precision float=w189:dbl[])
          n141 = call "DWE Error Notifier.vi"("Tab Control 3"=w180, "Tab num"=w181, "Errors 1"=w182) -> ()  [unwired: 8 in, 1 out]
          n142 = Bundle(w189, w188) -> (w192:cluster{dbl[], u16[]})  [unwired: 1 in]
          n143 = Bundle(w189, w187) -> (w191:cluster{dbl[], dbl[]})  [unwired: 1 in]
          n144 = Bundle(w189, w186) -> (w190:cluster{dbl[], dbl[]})  [unwired: 1 in]
          n145 = Build Array(w192, w191, w190) -> (→"Digital signals 7":cluster{dbl[], dbl[]}[])
          n146 = Bundle(w189, w195) -> (w198:cluster{dbl[], dbl[]})  [unwired: 1 in]
          n147 = Bundle(w189, w194) -> (w197:cluster{dbl[], dbl[]})  [unwired: 1 in]
          n148 = Bundle(w189, w193) -> (w196:cluster{dbl[], u16[]})  [unwired: 1 in]
          n149 = Bundle(w189, w199) -> (→"Current (mA) 7":cluster{dbl[], dbl[]})  [unwired: 1 in]
          n150 = Build Array(w198, w197, w196) -> (→"XY Graph 16":cluster{dbl[], dbl[]}[])
          "Errors 6" <- w182
        }
        frame 8 {
          n151 = To Double Precision Float(number=w221) -> (double precision float=w210:dbl[])
          n152 = call "DWE Error Notifier.vi"("Tab Control 3"=w201, "Tab num"=w202, "Errors 1"=w203) -> ()  [unwired: 8 in, 1 out]
          n153 = Bundle(w210, w209) -> (w213:cluster{dbl[], u16[]})  [unwired: 1 in]
          n154 = Bundle(w210, w208) -> (w212:cluster{dbl[], dbl[]})  [unwired: 1 in]
          n155 = Bundle(w210, w207) -> (w211:cluster{dbl[], dbl[]})  [unwired: 1 in]
          n156 = Bundle(w210, w220) -> (→"Current (mA) 8":cluster{dbl[], dbl[]})  [unwired: 1 in]
          n157 = Build Array(w213, w212, w211) -> (→"Digital signals 8":cluster{dbl[], dbl[]}[])
          n158 = Bundle(w210, w216) -> (w219:cluster{dbl[], dbl[]})  [unwired: 1 in]
          n159 = Bundle(w210, w215) -> (w218:cluster{dbl[], dbl[]})  [unwired: 1 in]
          n160 = Bundle(w210, w214) -> (w217:cluster{dbl[], u16[]})  [unwired: 1 in]
          n161 = Build Array(w219, w218, w217) -> (→"XY Graph 17":cluster{dbl[], dbl[]}[])
          "Errors 7" <- w203
        }
        frame 9 {
          n162 = To Double Precision Float(number=w242) -> (double precision float=w231:dbl[])
          n163 = call "DWE Error Notifier.vi"("Tab Control 3"=w222, "Tab num"=w223, "Errors 1"=w224) -> ()  [unwired: 8 in, 1 out]
          n164 = Bundle(w231, w230) -> (w234:cluster{dbl[], u16[]})  [unwired: 1 in]
          n165 = Bundle(w231, w229) -> (w233:cluster{dbl[], dbl[]})  [unwired: 1 in]
          n166 = Bundle(w231, w228) -> (w232:cluster{dbl[], dbl[]})  [unwired: 1 in]
          n167 = Bundle(w231, w241) -> (→"Current (mA) 9":cluster{dbl[], dbl[]})  [unwired: 1 in]
          n168 = Bundle(w231, w238) -> (w240:cluster{dbl[], dbl[]})  [unwired: 1 in]
          n169 = Bundle(w231, w237) -> (w239:cluster{dbl[], dbl[]})  [unwired: 1 in]
          n170 = Bundle(w231, w236) -> (w235:cluster{dbl[], u16[]})  [unwired: 1 in]
          n171 = Build Array(w234, w233, w232) -> (→"Digital signals 9":cluster{dbl[], dbl[]}[])
          n172 = Build Array(w240, w239, w235) -> (→"XY Graph 18":cluster{dbl[], dbl[]}[])
          "Errors 8" <- w224
        }
        frame 10 {
          n173 = To Double Precision Float(number=w263) -> (double precision float=w252:dbl[])
          n174 = call "DWE Error Notifier.vi"("Tab Control 3"=w243, "Tab num"=w244, "Errors 1"=w245) -> ()  [unwired: 8 in, 1 out]
          n175 = Bundle(w252, w251) -> (w255:cluster{dbl[], u16[]})  [unwired: 1 in]
          n176 = Bundle(w252, w250) -> (w254:cluster{dbl[], dbl[]})  [unwired: 1 in]
          n177 = Bundle(w252, w249) -> (w253:cluster{dbl[], dbl[]})  [unwired: 1 in]
          n178 = Build Array(w255, w254, w253) -> (→"Digital signals 10":cluster{dbl[], dbl[]}[])
          n179 = Bundle(w252, w262) -> (→"Current (mA) 10":cluster{dbl[], dbl[]})  [unwired: 1 in]
          n180 = Bundle(w252, w261) -> (w258:cluster{dbl[], dbl[]})  [unwired: 1 in]
          n181 = Bundle(w252, w260) -> (w257:cluster{dbl[], dbl[]})  [unwired: 1 in]
          n182 = Bundle(w252, w259) -> (w256:cluster{dbl[], u16[]})  [unwired: 1 in]
          n183 = Build Array(w258, w257, w256) -> (→"XY Graph 19":cluster{dbl[], dbl[]}[])
          "Errors 9" <- w245
        }
      }
    }
    "Day" <- w25
    n184 = Wait (ms)(milliseconds to wait=u32 30000) -> ()  [unwired: 1 out]
    "Iteration" <- w26
  }
